vi "Hermitian Conjugate Validation.vi"(7 "FFT Length":u16, 8 "Input Valid":bool, 9 "FFT Input Index":fxp<+,4,4>, 10 "FFT Calc Done":bool=TRUE, 11 "FFT Data":fxp<+,4,4>) -> (0 "Output Data Valid":bool, 1 "FFT Output Index":u16, 2 "FFT Stream1":T1, 3 "FFT Stream 0":T1)   [LabVIEW 2011]
doc: "This VI calculates Hermitian Conjugate of a Complex FFT Stream."
uses:
  <vilib>/rvi/XilinxIP/XIPIN_XNode/niFpgaXIPIN.xnode
  Users/kvemishe/AppData/Local/Temp/Untitled 1/Block Memory Generator/GenFiles66632D5441FD36EB00E2D1A20BC15D2B/Block_Memory_GeneratorSimFiles/Block_Memory_Generator_A99B750F4A20A6B4EECE81BFE09EA886.dll
  <vilib>/rvi/IPIntegrationNode/IPINode_Xnode/niFpgaIPINode.xnode
  <vilib>/rvi/IPIntegrationNode/IPINode_Utilities/niFpgaIPINodeSimCore.vi
  FFT/FFT subVIs/FFT RealIm Type.ctl
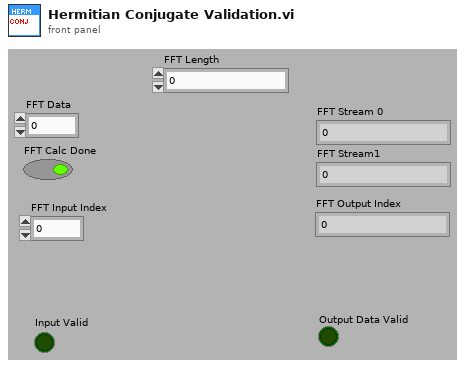
[diagram p1: front panel]
types:
  T1 = typedef "FFT RealIm Type.ctl" = fxp<+,32,32>
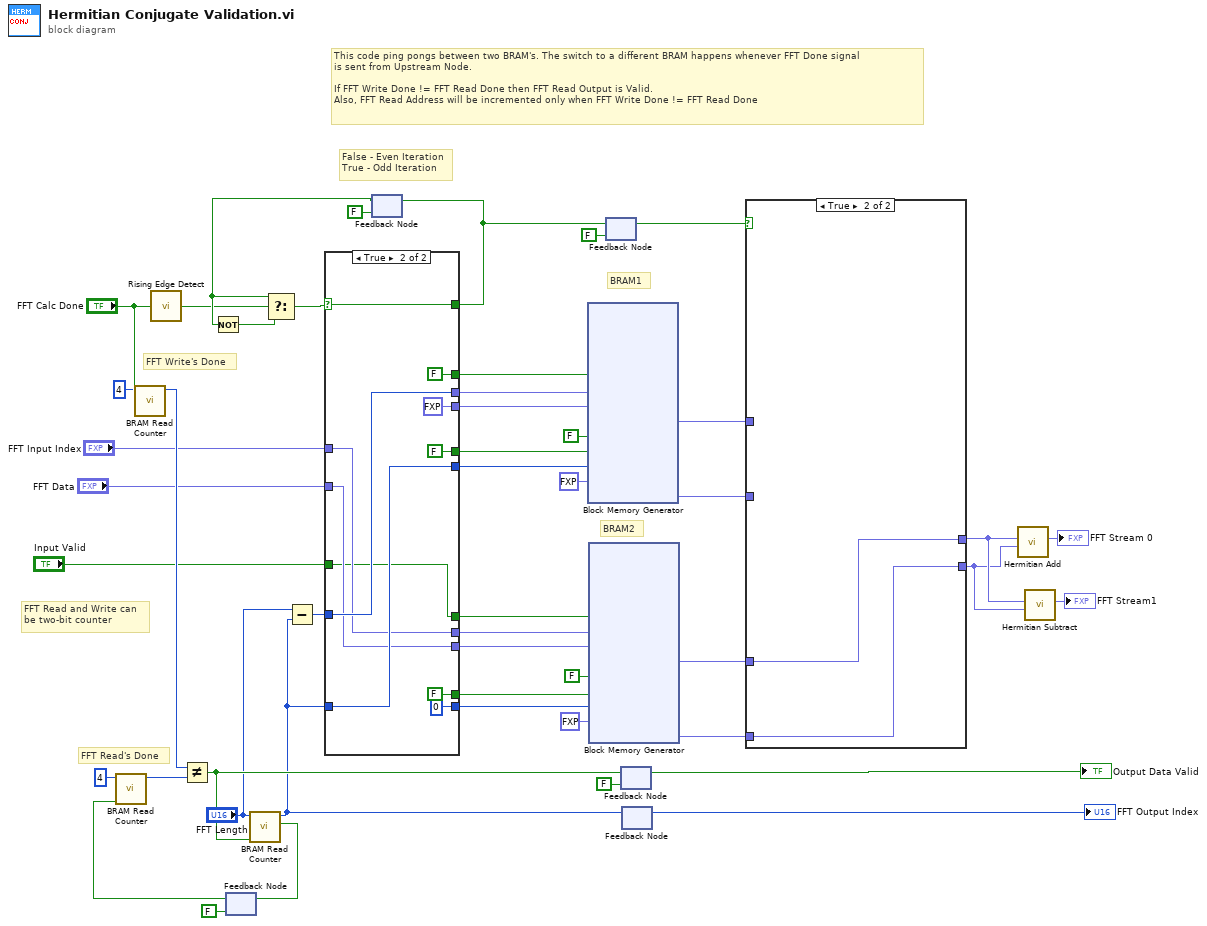
[diagram p0: block diagram]
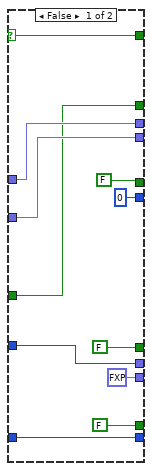
[diagram p3: hidden frame]
diagram:
  # "FFT Read and Write can\nbe two-bit counter"
  # "FFT Write's Done"
  # "FFT Read's Done"
  # "This code ping pongs between two BRAM's. The switch to a different BRAM happens whenever FFT Done signal\nis sent from Upstream Node.\n\nIf FFT Write Done != FFT Read Done then FFT Read Output is Valid.\nAlso, FFT Read Address will be incremented only when FFT Write Done != FFT Read Done"
  # "BRAM2"
  # "BRAM1"
  # "False - Even Iteration\nTrue - Odd Iteration"
  n1 = call "BRAM Read Counter.vi"("INC?"="FFT Calc Done", "rollover"=u16 4) -> ("count"=w31:u16)  [unwired: 8 in, 1 out]
  n2 = call <userlib>:"Rising Edge Detect.vi"("signal"="FFT Calc Done") -> ("edge detected"=w36:bool)  [unwired: 14 in]
  n3 = feedback #1(FALSE ("tc")) -> (w27:bool)
  n4 = call "BRAM Read Counter.vi"("INC?"=w27, "rollover"=u16 4) -> ("count"=w30:u16)  [unwired: 8 in, 1 out]
  n5 = Not Equal?(x=w31, y=w30) -> (x != y?=w26:bool)
  n6 = call "BRAM Read Counter.vi"("INC?"=w26, "rollover"="FFT Length") -> ("tc"=w29:bool, "count"=w1:u16)  [unwired: 8 in]
  n7 = feedback-in #1(w29) -> ()
  n8 = Subtract(x="FFT Length", y=w1) -> (x-y=w2:u16)
  n9 = feedback #2(FALSE) -> (w40:bool)
  n10 = Not(x=w40) -> (.not. x?=w39:bool)
  n11 = Select(t=w40, s=w36, f=w39) -> (s? t:f=w38:bool)
  n12 = case shown="True" w38 {
    selector: w38 -> [w56 w67]
    tunnel: [w49 FALSE] -> w48
    tunnel: [FALSE FALSE] -> w47
    tunnel: [FALSE w60] -> w46
    tunnel: [FALSE FALSE] -> w45
    tunnel: [w56 w67] -> w35
    tunnel: "FFT Input Index" -> [w55 w64]
    tunnel: [w55 w66] -> w17
    tunnel: w2 -> [w54 w66]
    tunnel: [w54 w64] -> w16
    tunnel: w1 -> [w53 w65]
    tunnel: [w53 u16 0] -> w14
    tunnel: [i16 0 w65] -> w13
    tunnel: [w51 fxp<+,4,4> 0.0 ("FFT Data")] -> w12
    tunnel: "FFT Data" -> [w51 w62]
    tunnel: [fxp<+,4,4> 0.0 ("FFT Data") w62] -> w10
    tunnel: "Input Valid" -> [w49 w60]
    frame False {
    }
    frame True {
    }
  }
  n13 = feedback-in #2(w35) -> ()
  n14 = xnode ("Block Memory Generator")("wea"=w48, "addra"=w17, "dina"=w12, "clkb"=FALSE, "web"=w47, "addrb"=w13, "dinb"=fxp<+,16,16> 0.0) -> ("douta"=w44:fxp<+,16,16>, "doutb"=w43:fxp<+,16,16>)
  n15 = xnode ("Block Memory Generator")("wea"=w46, "addra"=w16, "dina"=w10, "clkb"=FALSE, "web"=w45, "addrb"=w14, "dinb"=fxp<+,16,16> 0.0) -> ("douta"=w42:fxp<+,16,16>, "doutb"=w41:fxp<+,16,16>)
  n16 = feedback-in #3(w35) -> ()
  n17 = feedback #3(FALSE) -> (w33:bool)
  n18 = feedback-in #4(w26) -> ()
  n19 = feedback #4(FALSE) -> (→"Output Data Valid":bool)
  n20 = feedback #5() -> (→"FFT Output Index":u16)  [unwired: 1 in]
  n21 = feedback-in #5(w1) -> ()
  n22 = case shown="True" w33 {
    tunnel: w44 -> [w72 _]
    tunnel: w43 -> [w71 _]
    tunnel: w42 -> [_ w74]
    tunnel: w41 -> [_ w73]
    tunnel: [w72 w74] -> w22
    tunnel: [w71 w73] -> w21
    frame False {
    }
    frame True {
    }
  }
  n23 = call "Hermitian Add.vi"("Z2"=w21, "Z1"=w22) -> ("Zout"=→"FFT Stream 0":T1)  [unwired: 8 in, 1 out]
  n24 = call "Hermitian Subtract.vi"("Z2"=w21, "Z1"=w22) -> ("Zout"=→"FFT Stream1":T1)  [unwired: 8 in, 1 out]
